vi "Read Col.vi"(8 "error in (no error)":errorcluster, 11 "TreeEditCellMsg in":refnum<class "TreeEditCellMsg.lvclass">) -> (0 "error out":errorcluster, 2 "Col":i32, 3 "TreeEditCellMsg out":refnum<class "TreeEditCellMsg.lvclass">)   [LabVIEW 2020, in "ActorEvents.lvlib" / "TreeEditCellMsg.lvclass"]
uses:
  <vilib>/gpm_packages/@cs/mva-viewable/Source/ActorEvents/IEventAggregator Messages/TreeEditCellMsg/TreeEditCellMsg.lvclass
  <vilib>/gpm_packages/@cs/mva-viewable/Source/ActorEvents/IEventAggregator Messages/TreeEditCellMsg/TreeEditCellMsg.lvclass/TreeEditCellMsg.ctl
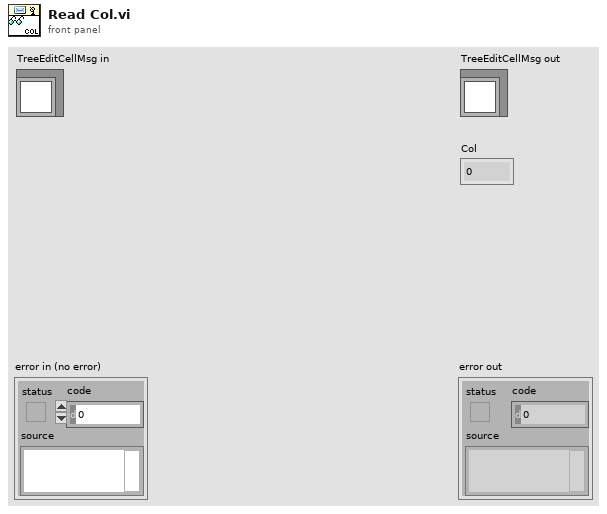
[diagram p1: front panel]
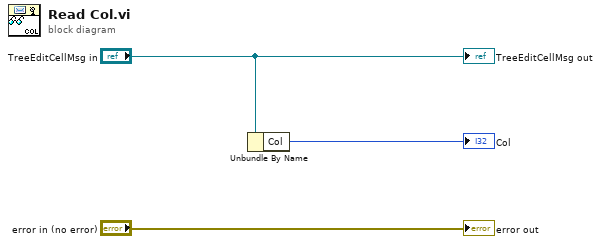
[diagram p0: block diagram]
diagram:
  n1 = Unbundle By Name("TreeEditCellMsg in") -> ("Col"=→"Col":i32)
  "error out" <- "error in (no error)"
  "TreeEditCellMsg out" <- "TreeEditCellMsg in"
